vi "Right_control.vi"(0 "Q_motor_In":refnum<queue>, 1 "V_TF_R":i32, 5 "Moter Cmd_param":T1, 7 "Param In":T2, 11 "에러 입력(에러 없음)":errorcluster) -> (4 "Q_motor_Out":refnum<queue>, 8 "Param out":T2, 15 "에러 출력":errorcluster)   [LabVIEW 2019]
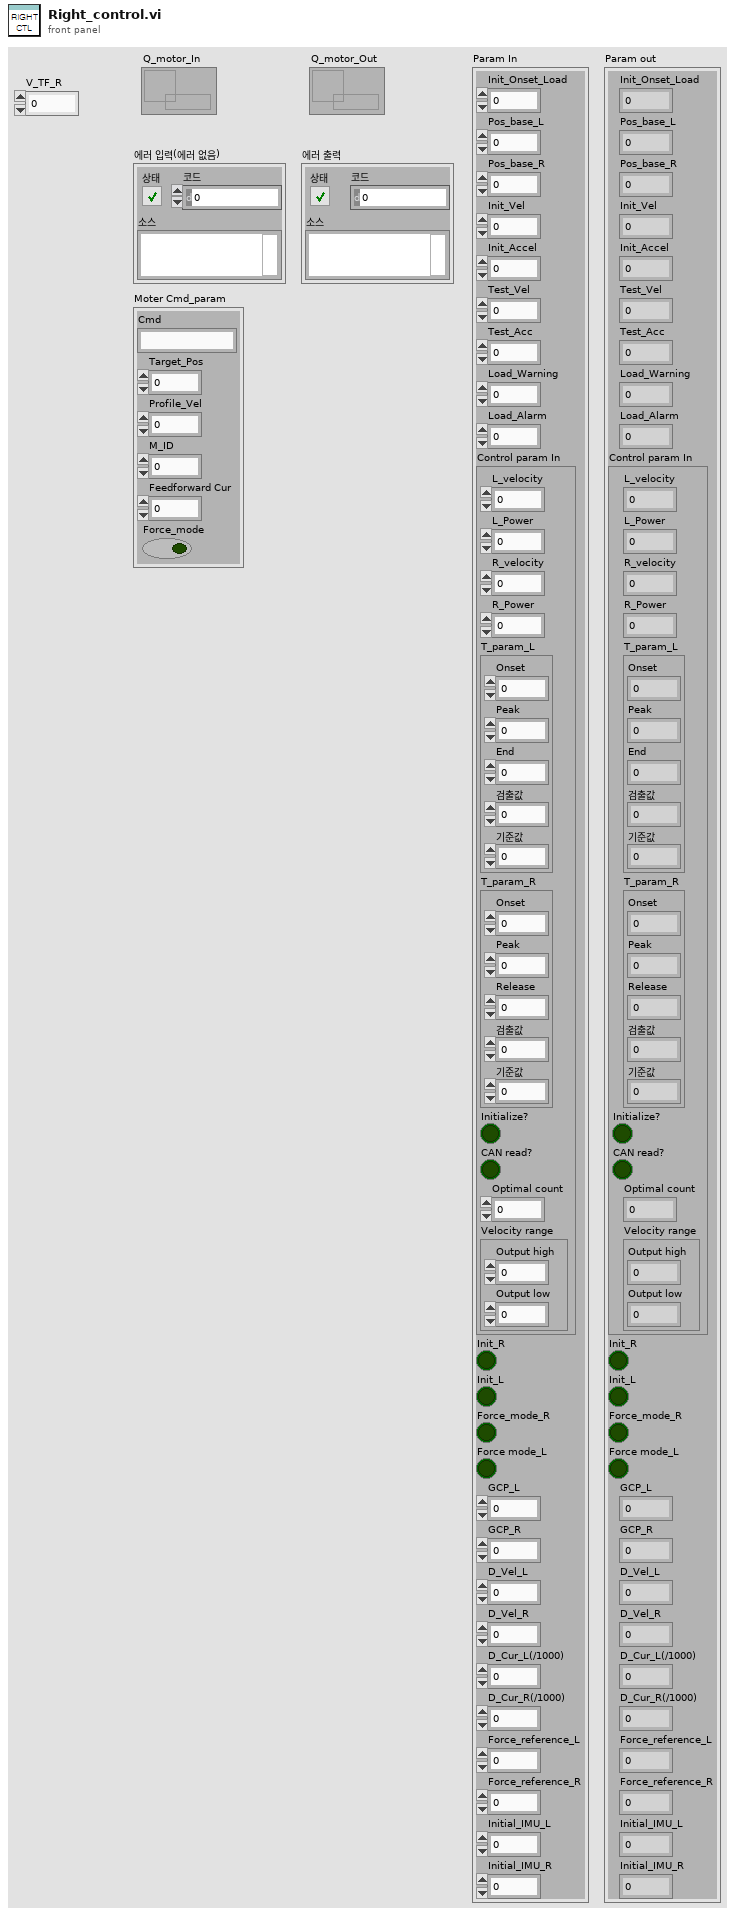
[diagram p1: front panel]
types:
  T1 = cluster{"Cmd":string, "Target_Pos":i32, "Profile_Vel":i32, "M_ID":u8, "Feedforward Cur":i16, "Force_mode":bool}
  T2 = cluster{"Init_Onset_Load":sgl, "Pos_base_L":sgl, "Pos_base_R":sgl, "Init_Vel":i32, "Init_Accel":u32, "Test_Vel":i32, "Test_Acc":u32, "Load_Warning":sgl, "Load_Alarm":sgl, "Control param In":cluster{"L_velocity":u32, "L_Power":sgl, "R_velocity":u32, "R_Power":sgl, "T_param_L":cluster{"Onset":sgl, "Peak":sgl, "End":sgl, "검출값":sgl, "기준값":sgl}, "T_param_R":cluster{"Onset":sgl, "Peak":sgl, "Release":sgl, "검출값":sgl, "기준값":sgl}, "Initialize?":bool, "CAN read?":bool, "Optimal count":i32, "Velocity range":cluster{"Output high":dbl, "Output low":dbl}}, "Init_R":bool, "Init_L":bool, "Force_mode_R":bool, "Force mode_L":bool, "GCP_L":sgl, "GCP_R":sgl, "D_Vel_L":sgl, "D_Vel_R":sgl, "D_Cur_L(/1000)":sgl, "D_Cur_R(/1000)":sgl, "Force_reference_L":sgl, "Force_reference_R":sgl, "Initial_IMU_L":sgl, "Initial_IMU_R":sgl}
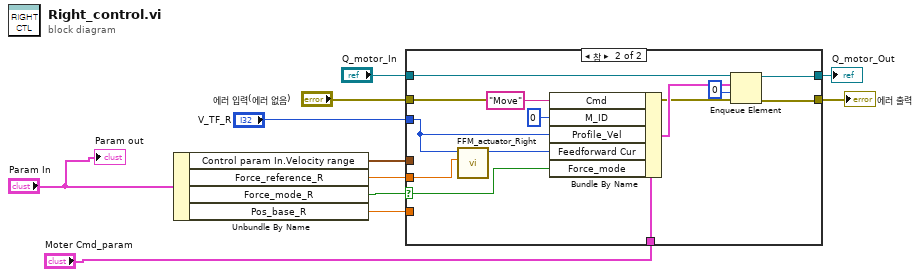
[diagram p0: block diagram]
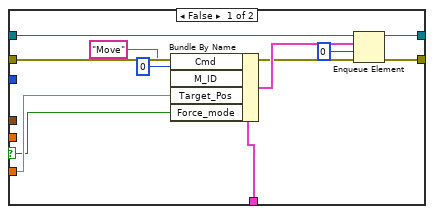
[diagram p2: hidden frame]
diagram:
  n1 = Unbundle By Name("Param In") -> ("Control param In.Velocity range"=w7:cluster{"Output high":dbl, "Output low":dbl}, "Force_reference_R"=w10:sgl, "Force_mode_R"=w9:bool, "Pos_base_R"=w11:sgl)
  n2 = case shown="참" w9 {
    selector: w9 -> [w14 w23]
    tunnel: w10 -> [_ w35]
    tunnel: w11 -> [w15 _]
    tunnel: "V_TF_R" -> [_ w32]
    tunnel: w7 -> [_ _]
    tunnel: "Moter Cmd_param" -> [w21 w29]
    tunnel: "Q_motor_In" -> [w19 w25]
    tunnel: "에러 입력(에러 없음)" -> [w18 w24]
    tunnel: [w17 w27] -> w5
    tunnel: [w16 w26] -> w2
    frame False {
      n3 = Bundle By Name(cluster=w21, "Cmd"="Move", "M_ID"=u8 0, "Target_Pos"=w15, "Force_mode"=w14) -> (w20:T1)
      n4 = Enqueue Element(queue=w19, element=w20, timeout in ms (-1)=0 ("타임아웃(ms) (-1)"), error in (no error)=w18) -> (queue out=w16:refnum<queue>, error out=w17:errorcluster)  [unwired: 1 out]
    }
    frame True {
      n5 = call "FFM_actuator_Right.vi"("Force_reference_R"=w35, "V_TF_R"=w32) -> ("숫자형"=w33:i16)  [unwired: 9 in]
      n6 = Bundle By Name(cluster=w29, "Cmd"="Move", "M_ID"=u8 0, "Profile_Vel"=w32, "Feedforward Cur"=w33, "Force_mode"=w23) -> (w28:T1)
      n7 = Enqueue Element(queue=w25, element=w28, timeout in ms (-1)=0 ("타임아웃(ms) (-1)"), error in (no error)=w24) -> (queue out=w26:refnum<queue>, error out=w27:errorcluster)  [unwired: 1 out]
    }
  }
  "에러 출력" <- w5
  "Q_motor_Out" <- w2
  "Param out" <- "Param In"
